vi "Cybersecurity_Game_v0.1.vi"() -> ()   [LabVIEW 2018]
panel:
  out "Available Coolant":dbl(slide) scale=0.0..10.0
  out "Active Control":bool
  in  "Button":bool
  in  "Stop Communication":bool
  in  "Cooling":dbl(slide) scale=0.0..10.0
  out "Color Box":u32(colorbox)
  out "Alerts":dbl
  out "Power":dbl(knob) scale=0.0..10000.0
  in  "Outgoing Messages":string
  out "Incoming Messages":string
  out "Temperature vs. Time":cluster{dbl[], dbl[]}(graph)
  # "Cybersecurity Game"
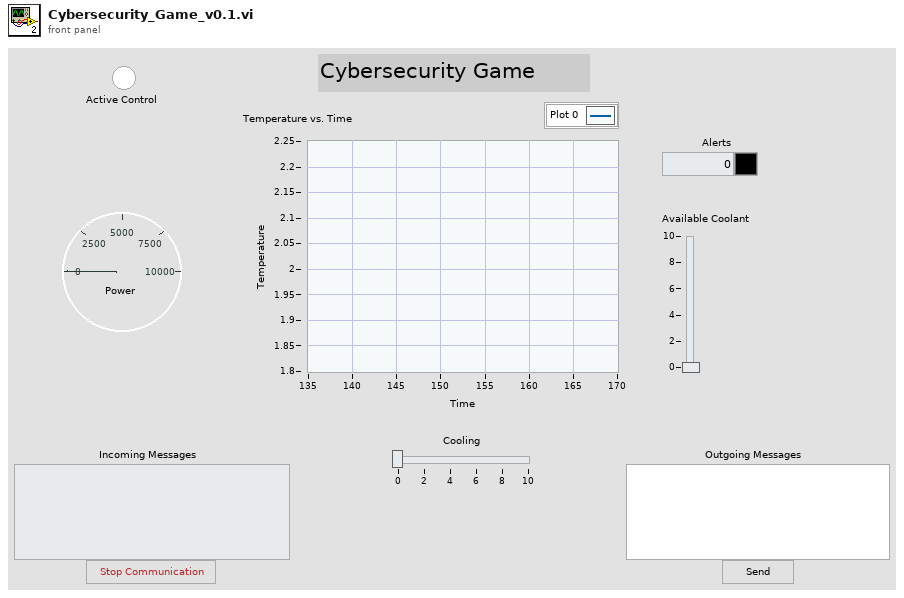
[diagram p1: front panel]
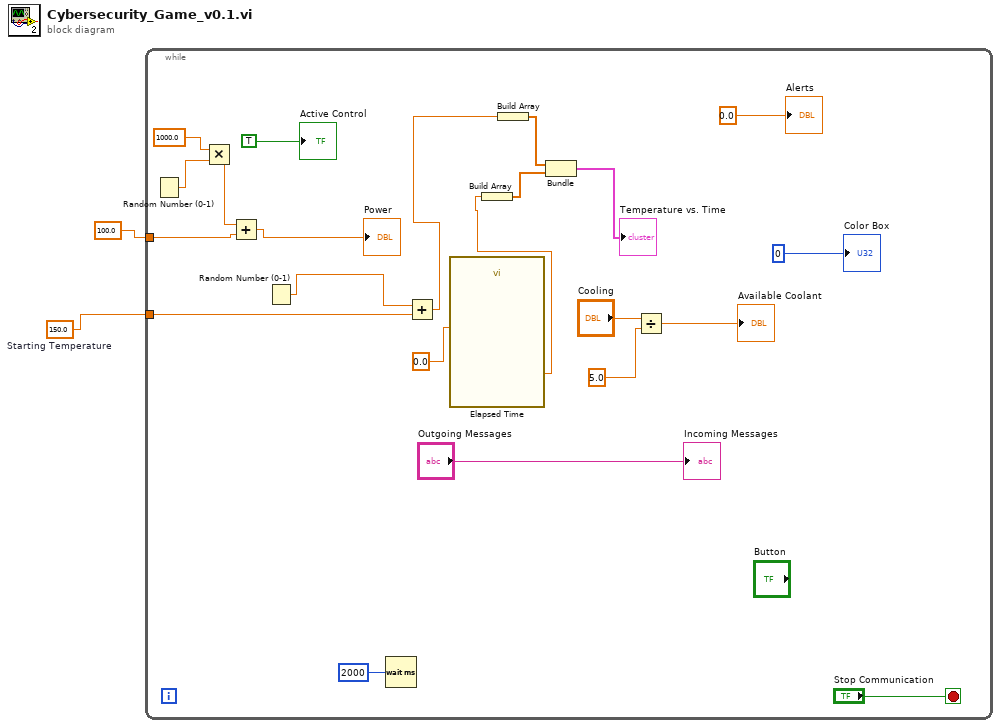
[diagram p0: block diagram]
diagram:
  w2 = 150.0  # Starting Temperature
  n1 = while {
    tunnel: w2 -> [w12]
    tunnel: 100.0 -> [w7]
    stop <- "Stop Communication" stop-if-true
    n2 = Random Number (0-1)() -> (number: 0 to 1=w5:dbl)
    n3 = Multiply(x=1000.0, y=w5) -> (x*y=w4:dbl)
    n4 = Add(x=w4, y=w7) -> (x+y=→"Power":dbl)
    n5 = Random Number (0-1)() -> (number: 0 to 1=w24:dbl)
    n6 = Wait (ms)(milliseconds to wait=u32 2000) -> ()  [unwired: 1 out]
    n7 = Add(x=w24, y=w12) -> (x+y=w11:dbl)
    n8 = call "Elapsed Time"("Set Start Time (s)"=0.0) -> ("Elapsed Time (s)"=w10:dbl)  [unwired: 11 in, 7 out]
    n9 = Build Array(w10) -> (w9:dbl[])
    n10 = Build Array(w11) -> (w8:dbl[])
    n11 = Bundle(w8, w9) -> (→"Temperature vs. Time":cluster{dbl[], dbl[]})  [unwired: 1 in]
    n12 = Divide(x="Cooling", y=5.0) -> (x/y=→"Available Coolant":dbl)
    "Incoming Messages" <- "Outgoing Messages"
    "Alerts" <- 0.0
    "Color Box" <- u32 0
    "Active Control" <- TRUE
  }
